vi "Check STDF File Path.vi"(8 "error in (no error)":errorcluster, 11 "STDF Files":string[](array[string])) -> (0 "error out":errorcluster, 3 "STDF Files out":string[](array[string]))   [LabVIEW 2018, in "STDF File Parser.lvclass"]
uses:
  STDF File Parser.lvclass
  <vilib>/Utility/error.llb/Error Cluster From Error Code.vi
  <vilib>/ErrorRing/Error Ring.xnode
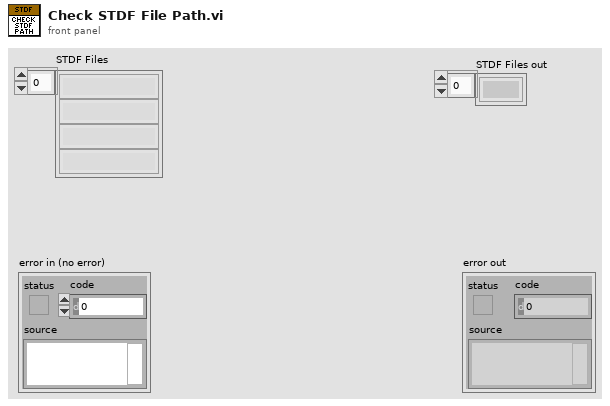
[diagram p1: front panel]
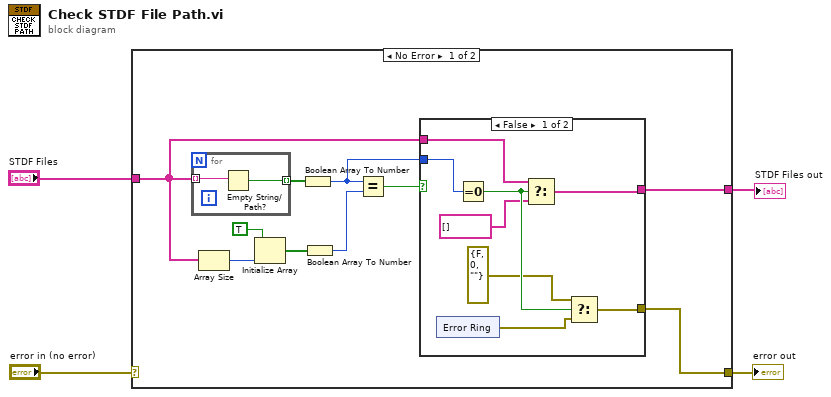
[diagram p0: block diagram]
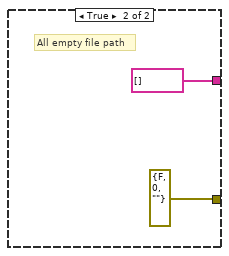
[diagram p2: hidden frame]
diagram:
  n1 = case shown="No Error" "error in (no error)" {
    selector: "error in (no error)" -> [_ w32]
    tunnel: [w6 w32] -> w3
    tunnel: "STDF Files" -> [w7 _]
    tunnel: [w5 _] -> w1
    frame No Error {
      n2 = for {
        tunnel: w7 -> [w31] mode=indexing
        tunnel: [w30] -> w11 mode=indexing
        n3 = Empty String/Path?(string/path=w31) -> (empty?=w30:bool)
      }
      n4 = Array Size(array=w7) -> (size(s)=w14:i32)
      n5 = Initialize Array(TRUE, w14) -> (w12:bool[])
      n6 = Boolean Array To Number(Boolean array=w11) -> (number=w8:u32)
      n7 = Boolean Array To Number(Boolean array=w12) -> (number=w10:u32)
      n8 = Equal?(x=w8, y=w10) -> (x = y?=w9:bool)
      n9 = case shown="False" w9 {
        tunnel: [w17 errorcluster {"status"=FALSE, "code"=0, "source"=""} ("error IO")] -> w6
        tunnel: w8 -> [w22 _]
        tunnel: w7 -> [w21 _]
        tunnel: [w15 string[] [] ("STDF Files")] -> w5
        frame False {
          n10 = xnode "Error Ring"() -> ("error out"=w18:errorcluster)
          n11 = Equal To 0?(x=w22) -> (x = 0?=w20:bool)
          n12 = Select(t=w21, s=w20, f=string[] []) -> (s? t:f=w15:string[])
          n13 = Select(t=errorcluster {"status"=FALSE, "code"=0, "source"=""} ("error IO"), s=w20, f=w18) -> (s? t:f=w17:errorcluster)
        }
        frame True {
          # "All empty file path"
        }
      }
    }
    frame Error {
    }
  }
  "error out" <- w3
  "STDF Files out" <- w1
